vi "temperature indicator.vi"() -> ()   [LabVIEW 2020]
panel:
  out "Temp 2":dbl
  out "Meter 2":dbl(knob) scale=-10.0..100.0
  out "moderate":bool
  out "Low Temp":bool
  out "High Temp":bool
  in  "Slide 2":dbl(slide) scale=-10.0..100.0
  in  "stop":bool
  # "VI Code to indicate  the\nchange in temperature"
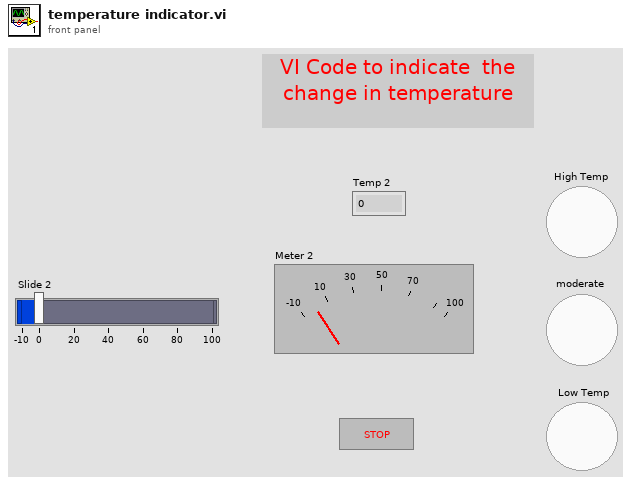
[diagram p1: front panel]
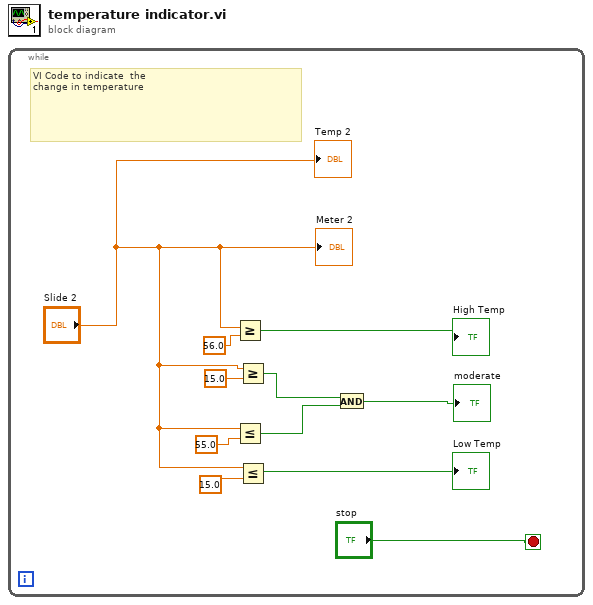
[diagram p0: block diagram]
diagram:
  n1 = while {
    stop <- "stop" stop-if-true
    # "VI Code to indicate  the\nchange in temperature"
    n2 = Greater Or Equal?(x="Slide 2", y=56.0) -> (x >= y?=→"High Temp":bool)
    n3 = Less Or Equal?(x="Slide 2", y=55.0) -> (x <= y?=w6:bool)
    n4 = Greater Or Equal?(x="Slide 2", y=15.0) -> (x >= y?=w5:bool)
    n5 = Less Or Equal?(x="Slide 2", y=15.0) -> (x <= y?=→"Low Temp":bool)
    n6 = And(x=w5, y=w6) -> (x .and. y?=→"moderate":bool)
    "Meter 2" <- "Slide 2"
    "Temp 2" <- "Slide 2"
  }
